vi "Acquire.vi"(8 "error in (no error)":errorcluster, 11 "Acquisition in":refnum<class "Acquisition.lvclass">) -> (0 "error out":errorcluster, 3 "Acquisition out":refnum<class "Acquisition.lvclass">)   [LabVIEW 2020, in "Acquisition.lvlib" / "Acquisition.lvclass"]
uses:
  Acquisition.lvclass
  C:/Program Files (x86)/National Instruments/LabVIEW 2020/vi.lib/ActorFramework/Actor/Actor.lvclass
  <vilib>/ActorFramework/Actor/Actor.lvclass/Actor.ctl
  Acquisition.lvclass/Acquisition.ctl
  UI Messages/Update Graph Msg/Update Graph Msg.lvclass/Update Graph Msg.ctl
  <vilib>/ActorFramework/Message Enqueuer/Message Enqueuer.lvclass/Message Enqueuer.ctl
  <vilib>/ActorFramework/Message Enqueuer/Enqueue.vi
  UI Messages/Update Graph Msg/Update Graph Msg.lvclass
  C:/Program Files (x86)/National Instruments/LabVIEW 2020/vi.lib/ActorFramework/Message/Message.lvclass
  <vilib>/ActorFramework/Message Priority Queue/Priority Enqueue.vi
  <vilib>/ActorFramework/Actor/Actor.lvclass
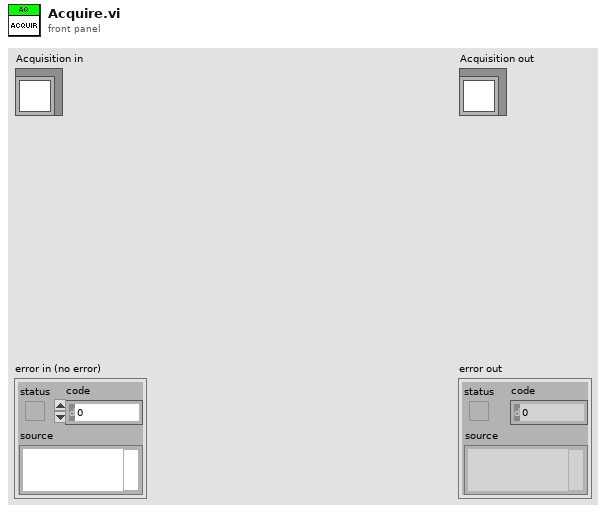
[diagram p1: front panel]
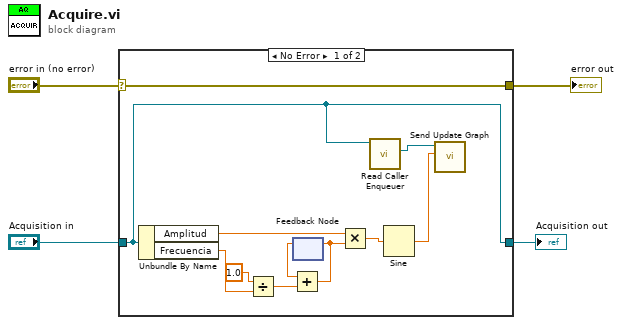
[diagram p0: block diagram]
diagram:
  n1 = case shown="No Error" "error in (no error)" {
    selector: "error in (no error)" -> [w15 w17]
    tunnel: [w15 w17] -> w3
    tunnel: [w7 w16] -> w1
    tunnel: "Acquisition in" -> [w7 w16]
    frame No Error {
      n2 = Unbundle By Name(w7) -> ("Amplitud"=w11:dbl, "Frecuencia"=w10:dbl)
      n3 = Divide(x=1.0 ("y"), y=w10) -> (x/y=w8:dbl)
      n4 = feedback #1() -> (w14:dbl)  [unwired: 1 in]
      n5 = Add(x=w14, y=w8) -> (x+y=w13:dbl)
      n6 = feedback-in #1(w13) -> ()
      n7 = Multiply(x=w11, y=w13) -> (x*y=w12:dbl)
      n8 = call <vilib>:"Read Caller Enqueuer.vi"("Actor"=w7) -> ("Caller Enqueuer"=w6:refnum<class "Message Enqueuer.lvclass">)  [unwired: 10 in]
      n9 = Sine(x=w12) -> (sin(x)=w5:dbl)
      n10 = call "Send Update Graph.vi"("Data"=w5, "Message Enqueuer"=w6) -> ()  [unwired: 8 in, 2 out]
    }
    frame Error {
    }
  }
  "error out" <- w3
  "Acquisition out" <- w1
